vi "Read XBox Buttons.vi"(8 "error in (no error)":errorcluster, 11 "XBoxController in":refnum<class "XBoxController.lvclass">) -> (0 "error out":errorcluster, 2 "XBox Buttons":T1, 3 "XBoxController out":refnum<class "XBoxController.lvclass">)   [LabVIEW 2013, in "XBoxController.lvclass"]
uses:
  XBoxController.lvclass
  Xbox Buttons.ctl
  XBoxController.lvclass/XBoxController.ctl
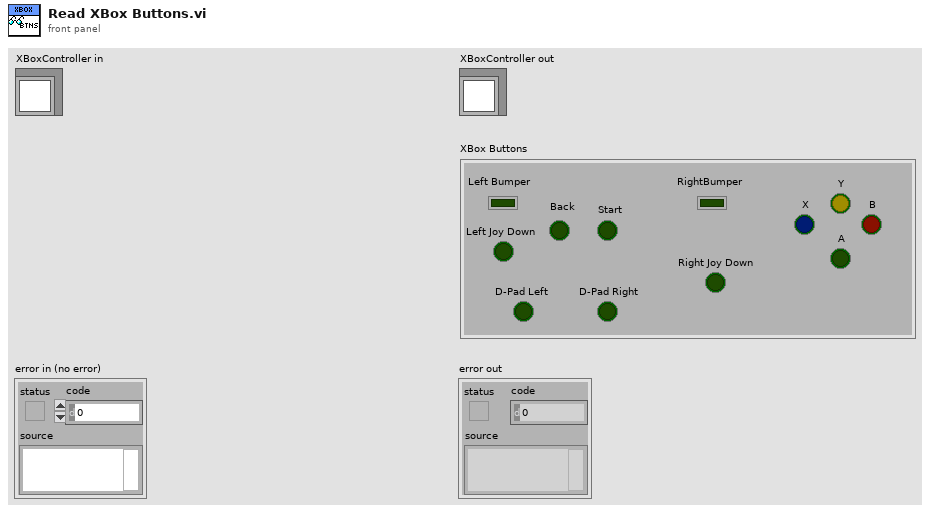
[diagram p1: front panel]
types:
  T1 = typedef "XBoxController.lvclass/Xbox Buttons.ctl" = cluster{"RightBumper":bool, "Left Bumper":bool, "Left Joy Down":bool, "Right Joy Down":bool, "Back":bool, "Start":bool, "D-Pad Left":bool, "D-Pad Right":bool, "Y":bool, "B":bool, "A":bool, "X":bool}
  T2 = typedef "WPI_JoystickDevRef.ctl" = cluster{"Device":T3}
  T3 = typedef "WPI_JoystickDeviceEnum.ctl" = enum16{"USB 1", "USB 2", "USB 3", "USB 4", "Kinect 1", "Kinect 2"}
  T4 = typedef "WPI_JoystickButtonState.ctl" = cluster{"Button 1":bool, "Button 2":bool, "Button 3":bool, "Button 4":bool, "Button 5":bool, "Button 6":bool, "Button 7":bool, "Button 8":bool, "Button 9":bool, "Button 10":bool, "Button 11":bool, "Button 12":bool}
  T5 = cluster{"axis 1 (x)":dbl, "axis 2 (y)":dbl, "axis 3 (throttle)":dbl, "axis 4":dbl, "axis 5":dbl, "axis 6":dbl}
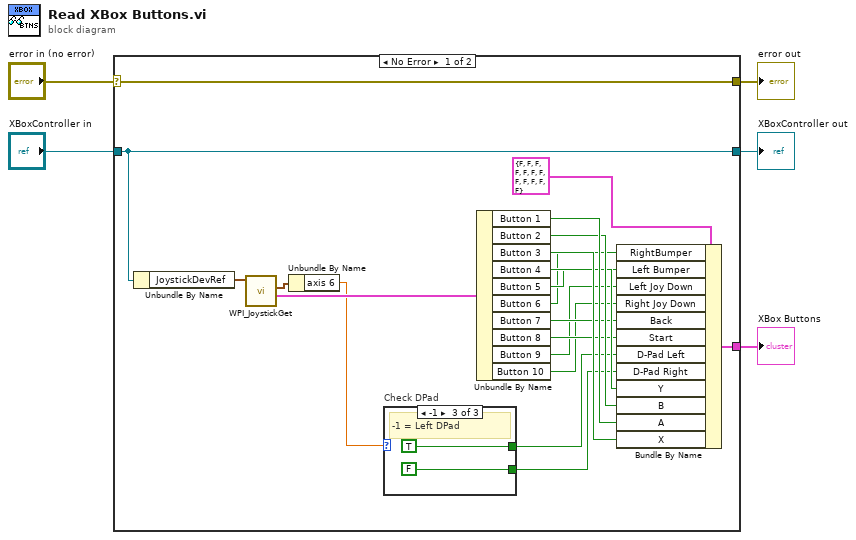
[diagram p0: block diagram]
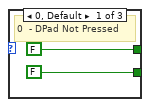
[diagram p2: hidden frame]
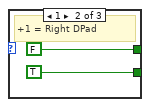
[diagram p3: hidden frame]
diagram:
  n1 = case shown="No Error" "error in (no error)" {
    selector: "error in (no error)" -> [w25 w32]
    tunnel: [w25 w32] -> w4
    tunnel: [w24 w33] -> w2
    tunnel: "XBoxController in" -> [w24 w33]
    tunnel: [w20 _] -> w1
    frame No Error {
      n2 = Unbundle By Name(w24) -> ("JoystickDevRef"=w23:T2)
      n3 = call <vilib>:"WPI_JoystickGet.vi"("JoystickDevRef"=w23) -> ("Buttons"=w22:T4, "Axes"=w9:T5)  [unwired: 4 in, 1 out]
      n4 = Unbundle By Name(w9) -> ("axis 6"=w8:dbl)
      n5 = case "Check DPad" shown="-1" w8 {
        tunnel: [FALSE FALSE TRUE] -> w7
        tunnel: [FALSE TRUE FALSE] -> w6
        frame 0, Default {
          # "0  - DPad Not Pressed"
        }
        frame 1 {
          # "+1 = Right DPad"
        }
        frame -1 {
          # "-1 = Left DPad"
        }
      }
      n6 = Unbundle By Name(w22) -> ("Button 1"=w19:bool, "Button 2"=w18:bool, "Button 3"=w17:bool, "Button 4"=w16:bool, "Button 5"=w15:bool, "Button 6"=w14:bool, "Button 7"=w13:bool, "Button 8"=w12:bool, "Button 9"=w11:bool, "Button 10"=w10:bool)
      n7 = Bundle By Name(cluster=T1 {"RightBumper"=FALSE, "Left Bumper"=FALSE, "Left Joy Down"=FALSE, "Right Joy Down"=FALSE, "Back"=FALSE, "Start"=FALSE, "D-Pad Left"=FALSE, "D-Pad Right"=FALSE, "Y"=FALSE, "B"=FALSE, "A"=FALSE, "X"=FALSE} ("XBox Buttons"), "RightBumper"=w14, "Left Bumper"=w15, "Left Joy Down"=w11, "Right Joy Down"=w10, "Back"=w13, "Start"=w12, "D-Pad Left"=w7, "D-Pad Right"=w6, "Y"=w16, "B"=w18, "A"=w19, "X"=w17) -> (w20:T1)
    }
    frame Error {
    }
  }
  "error out" <- w4
  "XBoxController out" <- w2
  "XBox Buttons" <- w1
